vi "PWM Counter.vi"(5 "Min Counter Value":u16, 6 "Waveform Generation Mode":fxp<+,2,2> format="%02b", 7 "Max Counter Value":u16, 10 "Enable":bool, 11 "Reset":bool) -> (1 "Counter is Min?":bool, 2 "Counter is Max?":bool, 3 "Counter Value":u16)   [LabVIEW 2016]
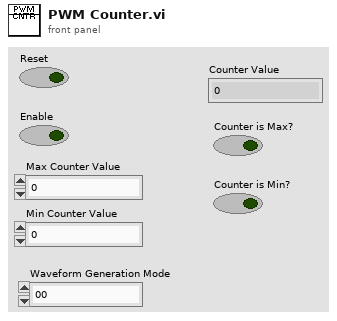
[diagram p1: front panel]
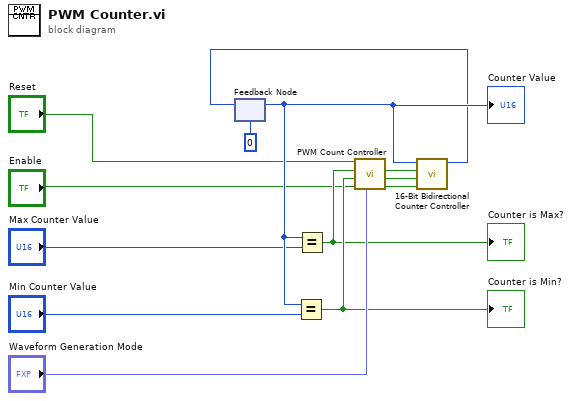
[diagram p0: block diagram]
diagram:
  n1 = feedback #1(u16 0 ("Value+")) -> (w12:u16)
  "Counter Value" <- w12
  n2 = Equal?(x=w12, y="Min Counter Value") -> (x = y?=w11:bool)
  "Counter is Min?" <- w11
  n3 = Equal?(x=w12, y="Max Counter Value") -> (x = y?=w10:bool)
  "Counter is Max?" <- w10
  n4 = call "PWM Count Controller.vi"("Waveform Generation Mode"="Waveform Generation Mode", "Enable In"="Enable", "Counter is Min?"=w11, "Counter is Max?"=w10, "Reset In"="Reset") -> ("Enable Out"=w5:bool, "Direction is Backward?"=w6:bool, "Reset Out"=w7:bool)  [unwired: 4 in]
  n5 = call "16-Bit Bidirectional Counter Controller.vi"("Enable"=w5, "Direction"=w6, "Reset"=w7, "Value"=w12) -> ("Value+"=w4:u16)  [unwired: 7 in]
  n6 = feedback-in #1(w4) -> ()
